vi "CloseDetector.vi"(0 "Averaging Size":i32=100, 1 "Initialize? (F)":bool, 2 "MaxVelosity":u16, 7 "ENCODER":i32) -> (4 "stop":bool)   [LabVIEW 2019, in "NeedleValve.lvclass"]
uses:
  NeedleValve_class/NeedleValve.lvclass
  <userlib>/_MGI/1D Array/MGI Average Type Enum.ctl
  <userlib>/_MGI/1D Array/MGI Running Average/MGI Running Average(DBL).vi
panel:
  out "enable stop":bool
  out "Waveform Chart":dbl(graph)
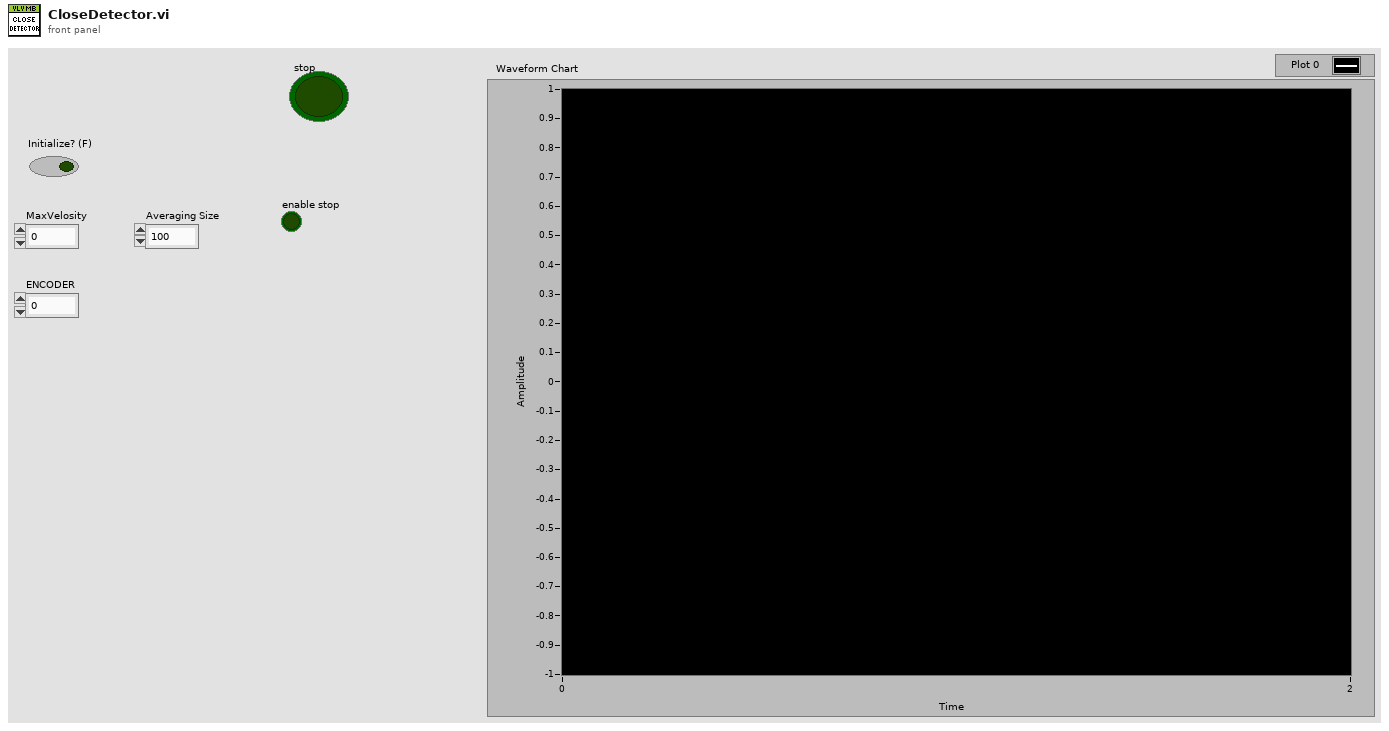
[diagram p1: front panel]
types:
  T1 = typedef "MGI Average Type Enum.ctl" = enum16{"Finite Impulse Response", "Infinite Impulse Response"}
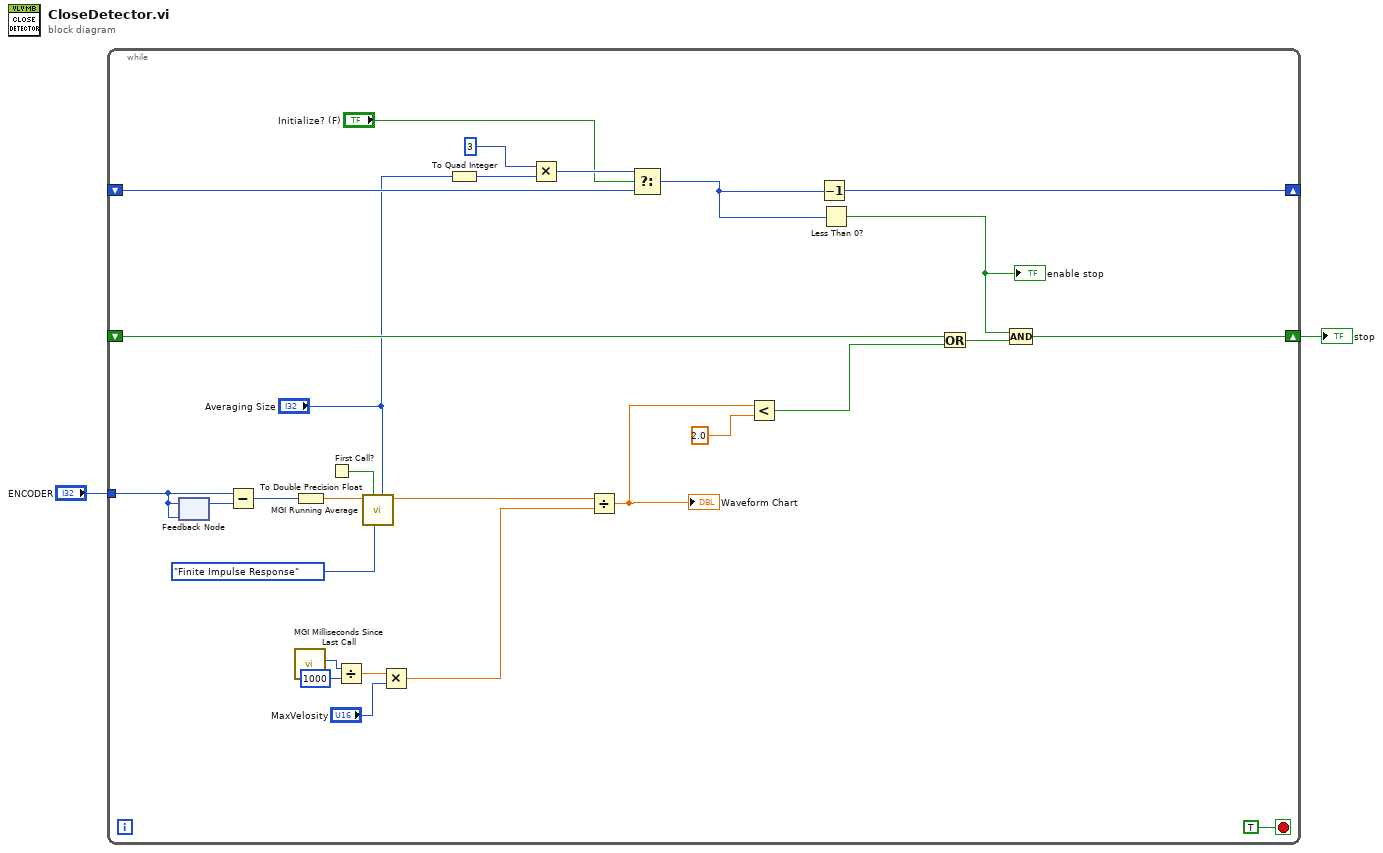
[diagram p0: block diagram]
diagram:
  n1 = while {
    tunnel: "ENCODER" -> [w4]
    shift-right: [w10] -> w1
    shift-left: _ -> [w19]
    shift-right: [w16] -> _
    shift-left: _ -> [w14]
    stop <- TRUE stop-if-true
    n2 = feedback #1(w4) -> (w30:i32)
    n3 = feedback-in #1(w4) -> ()
    n4 = Subtract(x=w4, y=w30) -> (x-y=w29:i32)
    n5 = call <userlib>:"MGI Milliseconds Since Last Call.vi"() -> ("ms"=w22:u32)  [unwired: 6 in, 1 out]
    n6 = To Double Precision Float(number=w29) -> (double precision float=w28:dbl)
    n7 = First Call?() -> (First Call?: T/F=w8:bool)
    n8 = Divide(x=w22, y=u32 1000) -> (x/y=w24:dbl)
    n9 = call-poly <userlib>:"MGI Running Average.vi"("Averaging Size"="Averaging Size", "Average Type(FIR)"=MGI_Average_Type_Enum."Finite Impulse Response", "Initialize? (F)"=w8, "Value"=w28) -> ("Average"=w21:dbl)  [unwired: 7 in]
    n10 = Multiply(x=w24, y="MaxVelosity") -> (x*y=w23:dbl)
    n11 = To Quad Integer(1:"Averaging Size") -> (0:w3:i64)
    n12 = Multiply(x=i64 3, y=w3) -> (x*y=w13:i64)
    n13 = Divide(x=w21, y=w23) -> (x/y=w5:dbl)
    "Waveform Chart" <- w5
    n14 = Select(t=w13, s="Initialize? (F)", f=w14) -> (s? t:f=w15:i64)
    n15 = Less?(x=w5, y=2.0) -> (x < y?=w18:bool)
    n16 = Decrement(x=w15) -> (x-1=w16:i64)
    n17 = Less Than 0?(x=w15) -> (x < 0?=w9:bool)
    "enable stop" <- w9
    n18 = Or(x=w19, y=w18) -> (x .or. y?=w11:bool)
    n19 = Compound Arithmetic op=AND(w9, w11) -> (w10:bool)
  }
  "stop" <- w1
